vi "draw_cellNum.vi"(7 "cell index":i32, 8 "error in":errorcluster, 9 "diameter (px)":i32=100, 10 "center (x,y)":i32[](array[numeric]), 11 "Image in":T2) -> (0 "error out":errorcluster, 3 "Image out":T2)   [LabVIEW 2015]
uses:
  <vilib>/vision/Image Controls.llb/IMAQ Image.ctl
panel:
  in  "Font, Size & Style":T1={"Desired Font (Application)"=enum."Application Font", "[User-specified Font]"={"Font Name"="Arial Black", "Size"=12, "Strikeout?"=FALSE, "Italic?"=FALSE, "Underline?"=FALSE, "Outline?"=FALSE, "Shadow?"=FALSE, "Bold?"=FALSE, "Rotation Angle"=0.0}, "Horizontal Alignment"=0, "Vertical Alignment"=0} {"Vertical Alignment" items=["Bottom", "Top", "Baseline"]; "Horizontal Alignment" items=["Left", "Center", "Right"]; "[User-specified Font]"."Rotation Angle" format="%.2f"}
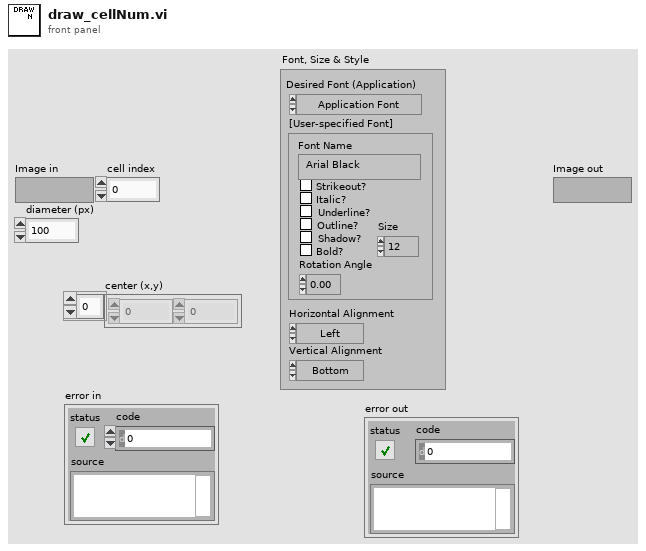
[diagram p1: front panel]
types:
  T1 = cluster{"Desired Font (Application)":enum16{"User-specified Font", "Application Font", "System Font", "Dialog Font"}, "[User-specified Font]":cluster{"Font Name":string, "Size":i16, "Strikeout?":bool, "Italic?":bool, "Underline?":bool, "Outline?":bool, "Shadow?":bool, "Bold?":bool, "Rotation Angle":dbl}, "Horizontal Alignment":i16, "Vertical Alignment":i16}
  T2 = typedef "IMAQ Image.ctl" = refnum<image>
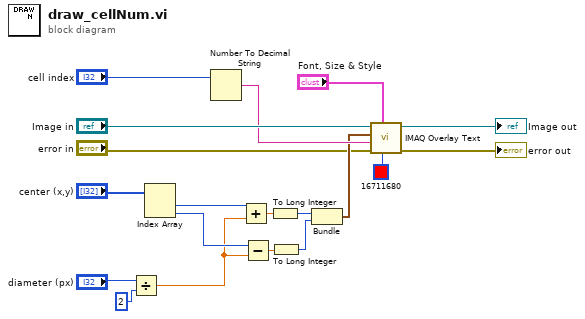
[diagram p0: block diagram]
diagram:
  n1 = Divide(x="diameter (px)", y=2) -> (x/y=w14:dbl)
  n2 = Index Array(array="center (x,y)") -> (element #1=w18:i32, element #2=w15:i32)  [unwired: 2 in]
  n3 = Number To Decimal String(number="cell index") -> (decimal integer string=w9:string)  [unwired: 1 in]
  n4 = Add(x=w18, y=w14) -> (x+y=w8:dbl)
  n5 = Subtract(x=w15, y=w14) -> (x-y=w7:dbl)
  n6 = To Long Integer(number=w8) -> (32bit integer=w6:i32)
  n7 = To Long Integer(number=w7) -> (32bit integer=w5:i32)
  n8 = Bundle(w6, w5) -> (w4:cluster{i32, i32})  [unwired: 1 in]
  n9 = call "IMAQ Overlay Text"("Text Color (black)"=u32 16711680, "Font, Size & Style"="Font, Size & Style", "error in (no error)"="error in", "String"=w9, "Origin"=w4, "Image"="Image in") -> ("error out"=→"error out":errorcluster, "Image Out"=→"Image out":T2)  [unwired: 4 in]
